vi "MyTest_getGPUphotons.vi"() -> ()   [LabVIEW 2018]
uses:
  <vilib>/addons/lvgpu/lvcuda/CUDA CDB Device Ptr/CUDA CDB Device Ptr.lvclass
  <vilib>/addons/lvgpu/lvcuda/CUDA DBL Device Ptr/CUDA DBL Device Ptr.lvclass
  <vilib>/addons/lvgpu/lvcuda/CUDA CDB Device Ptr/Prepare CUDA Device Ptr For Lock.vi
  <vilib>/addons/lvgpu/lvcuda/CUDA Context/Prepare CUDA Context For Lock.vi
  <vilib>/addons/lvgpu/lvcuda/CUDA DBL Device Ptr/Prepare CUDA Device Ptr For Lock.vi
  <vilib>/addons/lvgpu/lvcuda/CUDA U8 Device Ptr/Set CUDA Device Ptr Properties.vi
  <vilib>/addons/lvgpu/lvcuda/CUDA CDB Device Ptr/Get CUDA Device Ptr Properties.vi
  <vilib>/addons/lvgpu/lvcuda/CUDA Context/Prepare CUDA Context For Unlock.vi
  <vilib>/addons/lvgpu/lvcuda/CUDA CDB Device Ptr/Prepare CUDA Device Ptr For Unlock.vi
  <vilib>/addons/lvgpu/lvcuda.lvlib
  <vilib>/addons/lvgpu/lvcuda/CUDA Context/CUDA Context.lvclass
  <vilib>/addons/lvgpu/lvcuda/CUDA U8 Device Ptr/CUDA U8 Device Ptr.lvclass
panel:
  in  "error in":errorcluster
  out "error out":errorcluster
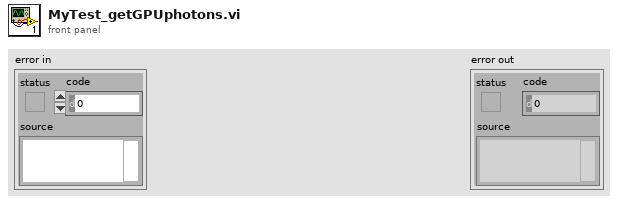
[diagram p1: front panel]
types:
  T1 = typedef "lvgpusdk.lvlib/GPU 1D DBL Array Data.lvclass/Array Data.ctl" = refnum<data-value>
  T2 = typedef "lvgpusdk.lvlib/GPU 1D CDB Array Data.lvclass/Array Data.ctl" = refnum<data-value>
  T3 = typedef "lvgpusdk.lvlib/GPU Custom Data.lvclass/Custom Data.ctl" = refnum<data-value>
  T4 = typedef "lvcuda.lvlib/CUDA Device Ptr (CUdeviceptr).ctl" = u64
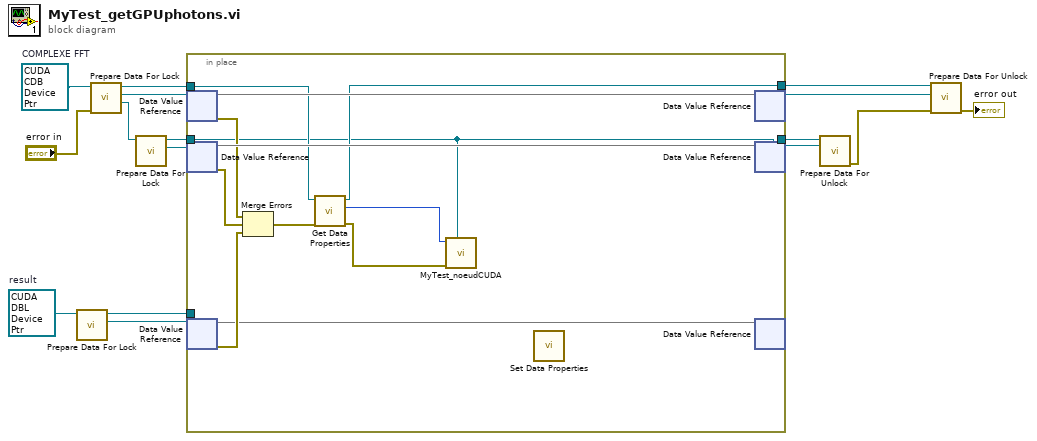
[diagram p0: block diagram]
diagram:
  w3 = refnum<class "CUDA DBL Device Ptr.lvclass"> refnum  # result
  w16 = refnum<class "CUDA CDB Device Ptr.lvclass"> refnum  # COMPLEXE FFT
  n1 = call-poly <vilib>:"Prepare Data For Lock.vi"("CUDA DBL Device Ptr in"=w3) -> ("CUDA DBL Device Ptr Data Reference"=w1:T1, "CUDA DBL Device Ptr out"=w2:refnum<class "CUDA DBL Device Ptr.lvclass">)  [unwired: 7 in, 2 out]
  n2 = call-poly <vilib>:"Prepare Data For Lock.vi"("error in"="error in", "CUDA CDB Device Ptr in"=w16) -> ("CUDA Context"=w9:refnum<class "CUDA Context.lvclass">, "CUDA CDB Device Ptr Data Reference"=w14:T2, "CUDA CDB Device Ptr out"=w15:refnum<class "CUDA CDB Device Ptr.lvclass">)  [unwired: 6 in, 1 out]
  n3 = call-poly <vilib>:"Prepare Data For Lock.vi"("CUDA Context in"=w9) -> ("CUDA Context Data Reference"=w7:T3, "CUDA Context out"=w8:refnum<class "CUDA Context.lvclass">)  [unwired: 8 in, 1 out]
  n4 = in-place {
    in-place-border: w15 -> [w26]
    in-place-border: [w25] -> w12
    in-place-border: w8 -> [w20]
    in-place-border: [w20] -> w5
    in-place-border: w2 -> [_]
    n5 = in-place-dvr #1(w14) -> (w28:cdb[], w23:errorcluster)
    n6 = in-place-dvr #2(w7) -> (w27:u8[], w24:errorcluster)
    n7 = in-place-dvr #3(w1) -> (w17:dbl[], w18:errorcluster)
    n8 = Merge Errors(w23, w24, w18) -> (w22:errorcluster)
    n9 = call-poly <vilib>:"Get Data Properties.vi"("error in"=w22, "CUDA CDB Device Ptr Data in"=w26) -> ("error out"=w21:errorcluster, "CDB *"=w19:T4, "CUDA CDB Device Ptr out"=w25:refnum<class "CUDA CDB Device Ptr.lvclass">)  [unwired: 5 in, 2 out]
    n10 = call "MyTest_noeudCUDA.vi"("CUDA Context out"=w20, "error IN"=w21, "CDB *"=w19) -> ()  [unwired: 9 in]
    n11 = call-poly <vilib>:"Set Data Properties.vi"() -> ()  [unwired: 10 in, 2 out]
    n12 = in-place-dvr #1(w28) -> (w13:T2)  [unwired: 1 out]
    n13 = in-place-dvr #2(w27) -> (w6:T3)  [unwired: 1 out]
    n14 = in-place-dvr #3(w17) -> ()  [unwired: 2 out]
  }
  n15 = call-poly <vilib>:"Prepare Data For Unlock.vi"("CUDA Context Data Reference"=w6, "CUDA Context in"=w5) -> ("error out"=w4:errorcluster)  [unwired: 8 in, 1 out]
  n16 = call-poly <vilib>:"Prepare Data For Unlock.vi"("error in"=w4, "CUDA CDB Device Ptr Data Reference"=w13, "CUDA CDB Device Ptr in"=w12) -> ("error out"=→"error out":errorcluster)  [unwired: 7 in, 1 out]
